vi "Host - Update Data (SubVI).vi"(8 "error in":errorcluster, 11 "Data in":T2={"VI References"=[], "Addresses"=[], "Pilot"=FALSE, "DO Data"=[], "Access Restricted?"=FALSE, "Pilot Control References"=[], "CoPilot Control References"=[], "cRIO Config"=[], "datalog Q"=refnum, "PS_P"={"AI"=[], "DI"=[], "DO"=[], "Serial"=[], "CPU"={"Total Load"=[], "Interrupt Load"=[], "Total Physical"=0.0, "Free Physical"=0.0, "Primary Disk Capacity"=0.0, "Primary Disk Free"=0.0}, "Stop"=FALSE, "DO Channel"=[]}, "PS_S"={"AI"=[], "DI"=[], "DO"=[], "Serial"=[], "CPU"={"Total Load"=[], "Interrupt Load"=[], "Total Physical"=0.0, "Free Physical"=0.0, "Primary Disk Capacity"=0.0, "Primary Disk Free"=0.0}, "Stop"=FALSE, "DO Channel"=[]}, "IDE_P"={"AI"=[], "DI"=[], "DO"=[], "Serial"=[], "CPU"={"Total Load"=[], "Interrupt Load"=[], "Total Physical"=0.0, "Free Physical"=0.0, "Primary Disk Capacity"=0.0, "Primary Disk Free"=0.0}, "Stop"=FALSE, "DO Channel"=[]}, "IDE_S"={"AI"=[], "DI"=[], "DO"=[], "Serial"=[], "CPU"={"Total Load"=[], "Interrupt Load"=[], "Total Physical"=0.0, "Free Physical"=0.0, "Primary Disk Capacity"=0.0, "Primary Disk Free"=0.0}, "Stop"=FALSE, "DO Channel"=[]}, "PDE_P"={"AI"=[], "DI"=[], "DO"=[], "Serial"=[], "CPU"={"Total Load"=[], "Interrupt Load"=[], "Total Physical"=0.0, "Free Physical"=0.0, "Primary Disk Capacity"=0.0, "Primary Disk Free"=0.0}, "Stop"=FALSE, "DO Channel"=[]}, "PDE_S"={"AI"=[], "DI"=[], "DO"=[], "Serial"=[], "CPU"={"Total Load"=[], "Interrupt Load"=[], "Total Physical"=0.0, "Free Physical"=0.0, "Primary Disk Capacity"=0.0, "Primary Disk Free"=0.0}, "Stop"=FALSE, "DO Channel"=[]}, "GUI References"={"Control Names"=[], "Control References"=[]}, "GUI Data"=[], "TCP - Serial"=[], "TCP-Serial Q"=refnum, "TCP Serial Ref"=[], "Data Sets"=[], "Last Data"=[], "Alarm Data"=[], "DI Data"=[], "Ack Data"=[], "Buzzer Data"=[], "Pilot DO"=[], "Co-Pilot DO"=[], "System Down?"=FALSE, "Log Data"=[], "Update Array"=[], "MCC Data Log"=[], "MCC Data Not"=refnum, "Thruster control"=[refnum, refnum, refnum, refnum, refnum, refnum, refnum, refnum, refnum], "waga notifier out"=refnum, "Wago  log"=[], "Thruster Cont"=[0.0, 0.0, 0.0, 0.0, 0.0, 0.0, 0.0, 0.0, 0.0], "Cam Cont"=[FALSE, FALSE, FALSE, FALSE, FALSE, TRUE], "PDE_P TH Cont"={"COM 10"=0.0, "COM 11"=0.0, "COM 12"=0.0, "COM 13"=0.0}, "PDE_S TH Cont"={"COM 10"=0.0, "COM 11"=0.0, "COM 12"=0.0, "COM 13"=0.0}} {"cRIO Config"."AI"."Interface Data"."Timing"."sample mode" items=["Finite Samples"=10178, "Continuous Samples"=10123, "Hardware Timed Single Point"=12522]; "cRIO Config"."Async"."Interface Data"."Data"."Minor Frame Count" min=5 max=8 step=1}) -> (0 "error out":errorcluster, 1 "# elements in queue":i32, 2 "output cluster":T1, 3 "Data out":T2={"VI References"=[], "Addresses"=[], "Pilot"=FALSE, "DO Data"=[], "Access Restricted?"=FALSE, "Pilot Control References"=[], "CoPilot Control References"=[], "cRIO Config"=[], "datalog Q"=refnum, "PS_P"={"AI"=[], "DI"=[], "DO"=[], "Serial"=[], "CPU"={"Total Load"=[], "Interrupt Load"=[], "Total Physical"=0.0, "Free Physical"=0.0, "Primary Disk Capacity"=0.0, "Primary Disk Free"=0.0}, "Stop"=FALSE, "DO Channel"=[]}, "PS_S"={"AI"=[], "DI"=[], "DO"=[], "Serial"=[], "CPU"={"Total Load"=[], "Interrupt Load"=[], "Total Physical"=0.0, "Free Physical"=0.0, "Primary Disk Capacity"=0.0, "Primary Disk Free"=0.0}, "Stop"=FALSE, "DO Channel"=[]}, "IDE_P"={"AI"=[], "DI"=[], "DO"=[], "Serial"=[], "CPU"={"Total Load"=[], "Interrupt Load"=[], "Total Physical"=0.0, "Free Physical"=0.0, "Primary Disk Capacity"=0.0, "Primary Disk Free"=0.0}, "Stop"=FALSE, "DO Channel"=[]}, "IDE_S"={"AI"=[], "DI"=[], "DO"=[], "Serial"=[], "CPU"={"Total Load"=[], "Interrupt Load"=[], "Total Physical"=0.0, "Free Physical"=0.0, "Primary Disk Capacity"=0.0, "Primary Disk Free"=0.0}, "Stop"=FALSE, "DO Channel"=[]}, "PDE_P"={"AI"=[], "DI"=[], "DO"=[], "Serial"=[], "CPU"={"Total Load"=[], "Interrupt Load"=[], "Total Physical"=0.0, "Free Physical"=0.0, "Primary Disk Capacity"=0.0, "Primary Disk Free"=0.0}, "Stop"=FALSE, "DO Channel"=[]}, "PDE_S"={"AI"=[], "DI"=[], "DO"=[], "Serial"=[], "CPU"={"Total Load"=[], "Interrupt Load"=[], "Total Physical"=0.0, "Free Physical"=0.0, "Primary Disk Capacity"=0.0, "Primary Disk Free"=0.0}, "Stop"=FALSE, "DO Channel"=[]}, "GUI References"={"Control Names"=[], "Control References"=[]}, "GUI Data"=[], "TCP - Serial"=[], "TCP-Serial Q"=refnum, "TCP Serial Ref"=[], "Data Sets"=[], "Last Data"=[], "Alarm Data"=[], "DI Data"=[], "Ack Data"=[], "Buzzer Data"=[], "Pilot DO"=[], "Co-Pilot DO"=[], "System Down?"=FALSE, "Log Data"=[], "Update Array"=[], "MCC Data Log"=[], "MCC Data Not"=refnum, "Thruster control"=[refnum, refnum, refnum, refnum, refnum, refnum, refnum, refnum, refnum], "waga notifier out"=refnum, "Wago  log"=[], "Thruster Cont"=[0.0, 0.0, 0.0, 0.0, 0.0, 0.0, 0.0, 0.0, 0.0], "Cam Cont"=[FALSE, FALSE, FALSE, FALSE, FALSE, TRUE], "PDE_P TH Cont"={"COM 10"=0.0, "COM 11"=0.0, "COM 12"=0.0, "COM 13"=0.0}, "PDE_S TH Cont"={"COM 10"=0.0, "COM 11"=0.0, "COM 12"=0.0, "COM 13"=0.0}} {"cRIO Config"."AI"."Interface Data"."Timing"."sample mode" items=["Finite Samples"=10178, "Continuous Samples"=10123, "Hardware Timed Single Point"=12522]; "cRIO Config"."Async"."Interface Data"."Data"."Minor Frame Count" min=5 max=8 step=1})   [LabVIEW 2021]
uses:
  Controls/Host - GUI Data Cluster.ctl
  Analog Output/Controls/AO JSON Data Cluster.ctl
  Analog Output/Controls/AO Interface Data Cluster.ctl
  Analog Output/Controls/AO Channel Configuration Cluster.ctl
  Analog Output/Controls/AO Timing Cluster.ctl
  Digital Output/Controls/DIO Configuration cluster.ctl
  Digital Output/Controls/DIO Interface Data.ctl
  Digital Output/SubVIs/Digital Dynamic Cluster.ctl
  Async JSON Cluster.ctl
  Async Interface Data Cluster.ctl
  Async Serial/Controls/Async Serial Configuration Cluster.ctl
  Async Serial/Controls/Async Frame Info Cluster.ctl
  Async Serial/Controls/Async Message Info Cluster.ctl
  Controls/Host Data Cluster.ctl
  Main Engine/Controls/Main Engine CPU Info.ctl
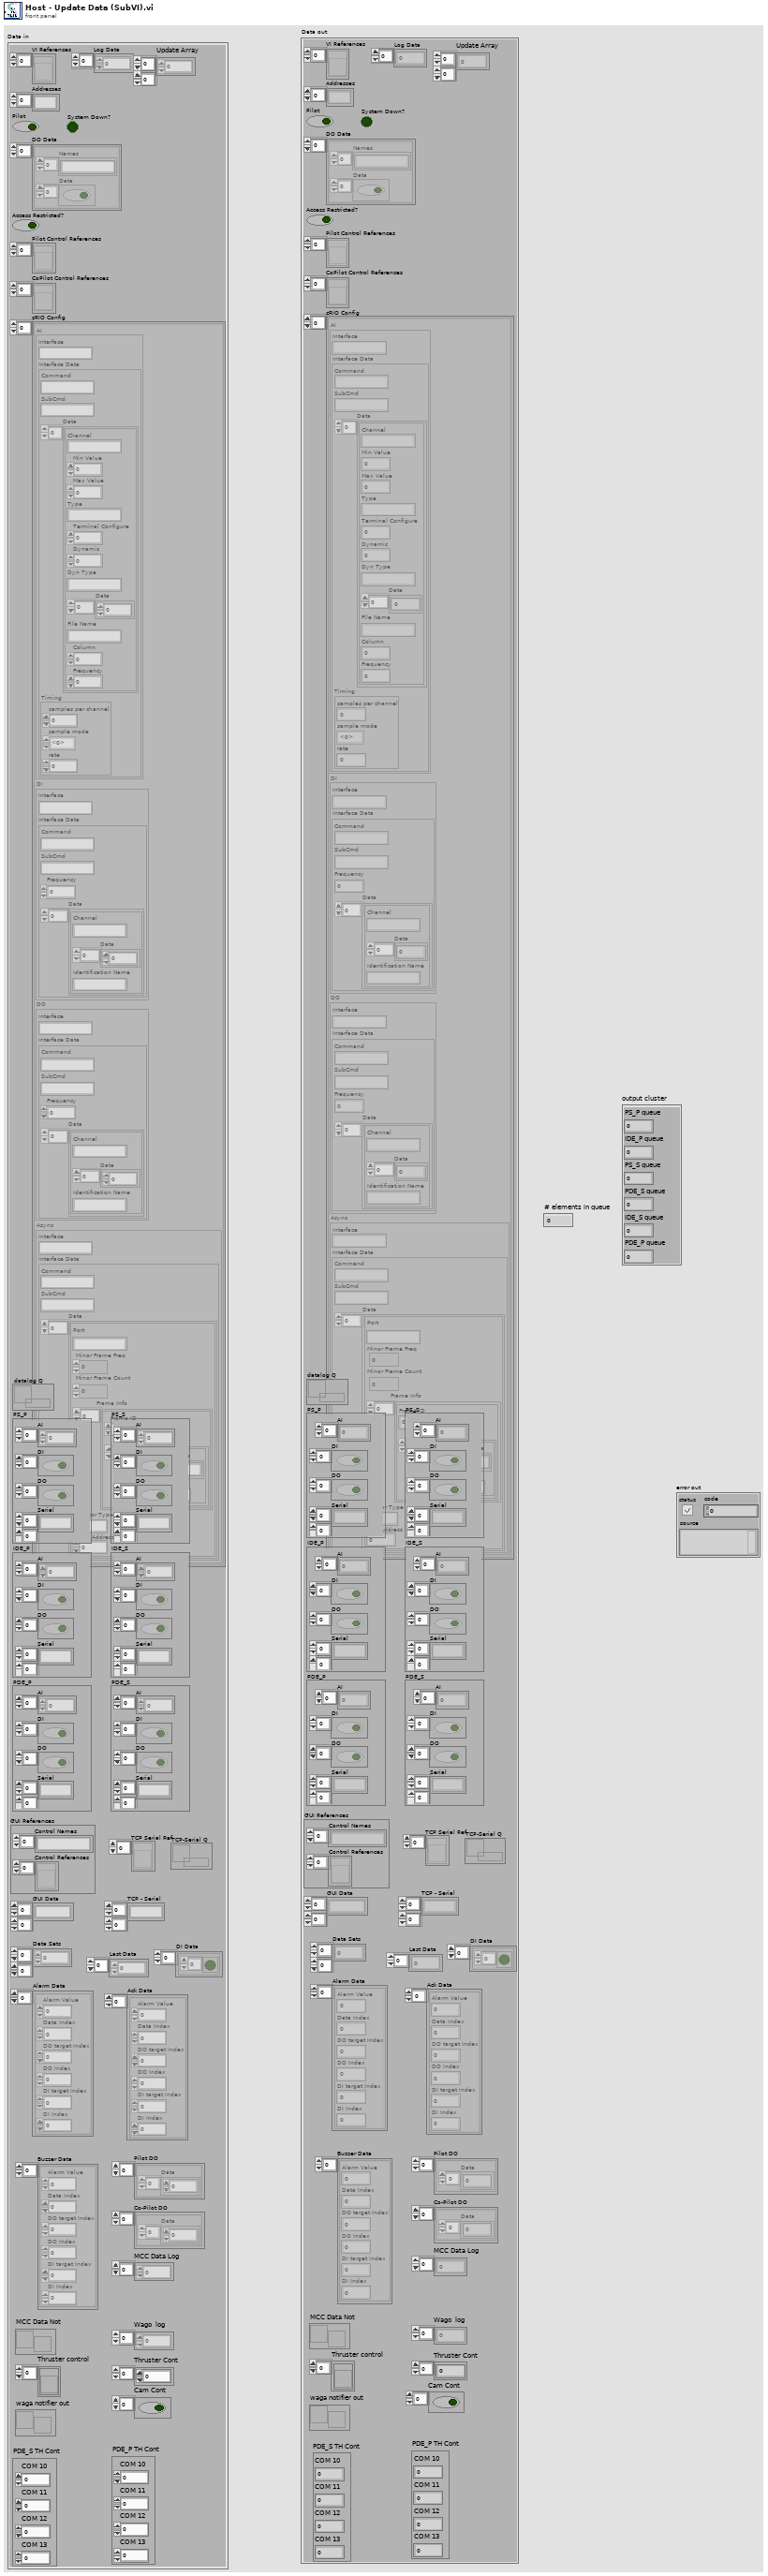
[diagram p1: front panel]
types:
  T1 = cluster{"PS_P queue":i32, "IDE_P queue":i32, "PS_S queue":i32, "PDE_S queue":i32, "IDE_S queue":i32, "PDE_P queue":i32}
  T2 = typedef "Host - GUI Data Cluster.ctl" = cluster{"VI References":refnum<vi>[], "Addresses":string[], "Pilot":bool, "DO Data":cluster{"Names":string[], "Data":bool[]}[], "Access Restricted?":bool, "Pilot Control References":refnum<vi>[], "CoPilot Control References":refnum<vi>[], "cRIO Config":cluster{"AI":T3, "DI":T7, "DO":T7, "Async":T10}[], "datalog Q":refnum<queue>, "PS_P":T15, "PS_S":T15, "IDE_P":T15, "IDE_S":T15, "PDE_P":T15, "PDE_S":T15, "GUI References":cluster{"Control Names":string[], "Control References":refnum<vi>[]}, "GUI Data":string[][], "TCP - Serial":string[][], "TCP-Serial Q":refnum<queue>, "TCP Serial Ref":refnum<vi>[], "Data Sets":dbl[][], "Last Data":dbl[], "Alarm Data":cluster{"Alarm Value":dbl, "Data Index":i32, "DO target Index":i32, "DO Index":i32, "DI target Index":i32, "DI Index":i32}[], "DI Data":cluster{bool[]}[], "Ack Data":cluster{"Alarm Value":dbl, "Data Index":i32, "DO target Index":i32, "DO Index":i32, "DI target Index":i32, "DI Index":i32}[], "Buzzer Data":cluster{"Alarm Value":dbl, "Data Index":i32, "DO target Index":i32, "DO Index":i32, "DI target Index":i32, "DI Index":i32}[], "Pilot DO":cluster{"Data":i32[]}[], "Co-Pilot DO":cluster{"Data":i32[]}[], "System Down?":bool, "Log Data":dbl[], "Update Array":i32[][], "MCC Data Log":dbl[], "MCC Data Not":refnum<notifier>, "Thruster control":refnum<vi>[], "waga notifier out":refnum<notifier>, "Wago  log":sgl[], "Thruster Cont":dbl[], "Cam Cont":bool[], "PDE_P TH Cont":cluster{"COM 10":dbl, "COM 11":dbl, "COM 12":dbl, "COM 13":dbl}, "PDE_S TH Cont":cluster{"COM 10":dbl, "COM 11":dbl, "COM 12":dbl, "COM 13":dbl}}
  T3 = typedef "AO JSON Data Cluster.ctl" = cluster{"Interface":string, "Interface Data":T4}
  T4 = typedef "AO Interface Data Cluster.ctl" = cluster{"Command":string, "SubCmd":string, "Data":T5[], "Timing":T6}
  T5 = typedef "AO Channel Configuration Cluster.ctl" = cluster{"Channel":string, "Min Value":dbl, "Max Value":dbl, "Type":string, "Terminal Configure":u16, "Dynamic":u8, "Dyn Type":string, "Data":dbl[], "File Name":string, "Column":i32, "Frequency":dbl}
  T6 = typedef "AO Timing Cluster.ctl" = cluster{"samples per channel":i32, "sample mode":i32, "rate":dbl}
  T7 = typedef "DIO Configuration cluster.ctl" = cluster{"Interface":string, "Interface Data":T8}
  T8 = typedef "DIO Interface Data.ctl" = cluster{"Command":string, "SubCmd":string, "Frequency":u16, "Data":T9[]}
  T9 = typedef "Digital Dynamic Cluster.ctl" = cluster{"Channel":string, "Data":u8[], "Identification Name":string}
  T10 = typedef "Async JSON Cluster.ctl" = cluster{"Interface":string, "Interface Data":T11}
  T11 = typedef "Async Interface Data Cluster.ctl" = cluster{"Command":string, "SubCmd":string, "Data":T12[]}
  T12 = typedef "Async Serial Configuration Cluster.ctl" = cluster{"Port":string, "Minor Frame Freq":u16, "Minor Frame Count":u16, "Frame Info":T13[], "Sensor Type":u16, "OIM Address":u16}
  T13 = typedef "Async Frame Info Cluster.ctl" = cluster{"Frame ID":u16, "Message Info":T14[]}
  T14 = typedef "Async Message Info Cluster.ctl" = cluster{"Message":u8[], "Message Name":string}
  T15 = typedef "Host Data Cluster.ctl" = cluster{"AI":dbl[], "DI":bool[], "DO":bool[], "Serial":string[][], "CPU":T16, "Stop":bool, "DO Channel":string[]}
  T16 = typedef "Main Engine CPU Info.ctl" = cluster{"Total Load":u32[], "Interrupt Load":u32[], "Total Physical":dbl, "Free Physical":dbl, "Primary Disk Capacity":dbl, "Primary Disk Free":dbl}
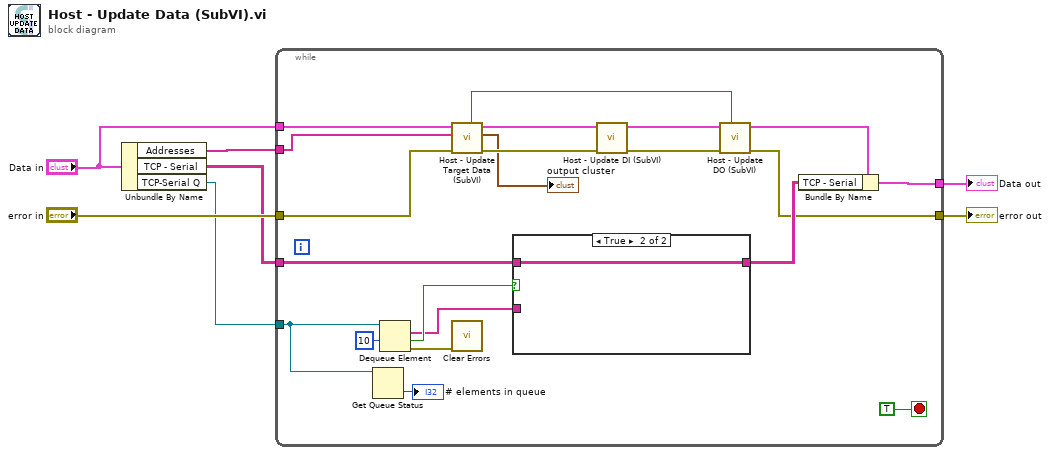
[diagram p0: block diagram]
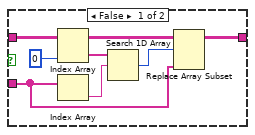
[diagram p2: hidden frame]
diagram:
  n1 = Unbundle By Name("Data in") -> ("Addresses"=w6:string[], "TCP - Serial"=w4:string[][], "TCP-Serial Q"=w1:refnum<queue>)
  n2 = while {
    tunnel: "error in" -> [w27]
    tunnel: w6 -> [w26]
    tunnel: [w14] -> w5
    tunnel: "Data in" -> [w24]
    tunnel: [w17] -> w3
    tunnel: w1 -> [w10]
    tunnel: w4 -> [w19]
    stop <- TRUE stop-if-true
    n3 = Get Queue Status(queue=w10) -> (# elements in queue=→"# elements in queue":i32)  [unwired: 2 in, 7 out]
    n4 = Dequeue Element(queue=w10, timeout in ms (-1)=10) -> (element=w18:string[], timed out?=w20:bool, error out=w21:errorcluster)  [unwired: 1 in, 1 out]
    n5 = call "Host - Update Target Data (SubVI).vi"("error in"=w27, "Addresses"=w26, "Data in"=w24) -> ("error out"=w13:errorcluster, "output cluster"=→"output cluster":T1, "Data out"=w12:T2, "DO Change?"=w11:bool)  [unwired: 5 in]
    n6 = call <vilib>:"Clear Errors.vi"("error in (no error)"=w21) -> ()  [unwired: 5 in, 2 out]
    n7 = case shown="True" w20 {
      tunnel: w19 -> [w31 w35]
      tunnel: w18 -> [w30 _]
      tunnel: [w28 w35] -> w16
      frame False {
        n8 = Index Array(array=w31, index (col)=0 ("disabled index (col)")) -> (element=w33:string[])  [unwired: 1 in]
        n9 = Index Array(array=w30) -> (element=w32:string)  [unwired: 1 in]
        n10 = Search 1D Array(1D array=w33, element=w32) -> (index of element=w29:i32)  [unwired: 1 in]
        n11 = Replace Array Subset(array=w31, new element=w30, index (row)=w29) -> (w28:string[][])  [unwired: 1 in]
      }
      frame True {
      }
    }
    n12 = call "Host - Update DI (SubVI).vi"("Data in"=w12) -> ("Data out"=w15:T2)  [unwired: 10 in]
    n13 = call "Host - Update DO (SubVI).vi"("DO Change?"=w11, "error in"=w13, "Data in"=w15) -> ("error out"=w14:errorcluster, "Data out"=w23:T2)  [unwired: 7 in]
    n14 = Bundle By Name(cluster=w23, "TCP - Serial"=w16) -> (w17:T2)
  }
  "error out" <- w5
  "Data out" <- w3
